vi "Host - Get Remote IO Module Data.vi"(8 "error in (no error)":errorcluster, 11 "Remote IO Mod IOVs":refnum<k21>[](array[refnum])) -> (0 "error out":errorcluster, 3 "Modules":T1[](array[typedef]))   [LabVIEW 2015, in "Scan Engine Custom Device.lvlib"]
uses:
  Scan Engine Custom Device.lvlib
  Type Defs/Host - Module.ctl
  <resource>/objmgr/IndComECAT.rc
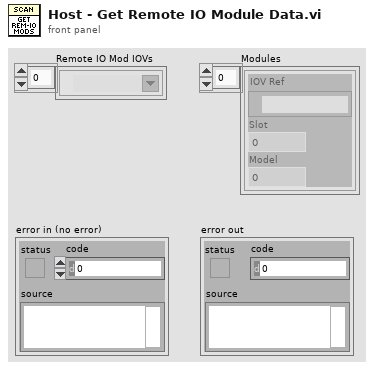
[diagram p1: front panel]
types:
  T1 = typedef "Scan Engine Custom Device.lvlib/Host - Module.ctl" = cluster{"IOV Ref":refnum<k21>, "Slot":u32, "Model":u32}
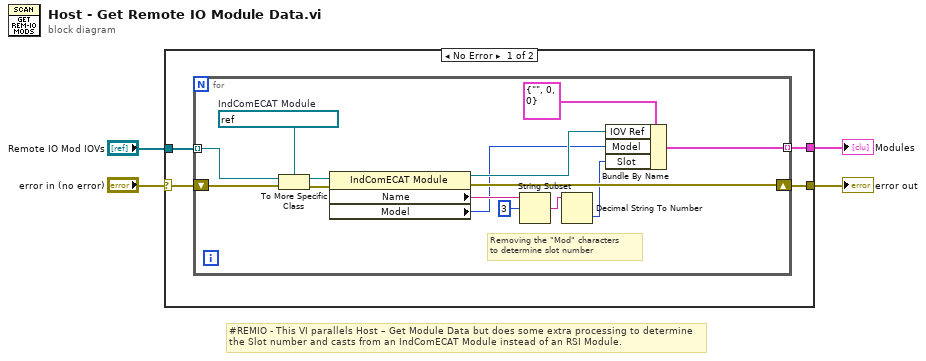
[diagram p0: block diagram]
diagram:
  # "#REMIO - This VI parallels Host – Get Module Data but does some extra processing to determine the Slot number and casts from an IndComECAT Module instead of an RSI Module."
  n1 = case shown="No Error" "error in (no error)" {
    selector: "error in (no error)" -> [w6 w23]
    tunnel: [w8 _] -> w4
    tunnel: [w7 w23] -> w3
    tunnel: "Remote IO Mod IOVs" -> [w5 _]
    frame No Error {
      n2 = for {
        shift-right: [w14] -> w7
        shift-left: w6 -> [w13]
        tunnel: [w22] -> w8 mode=indexing
        tunnel: w5 -> [w16] mode=indexing
        w15 = refnum<k21> refnum  # IndComECAT Module
        # "Removing the \"Mod\" characters\nto determine slot number"
        n3 = To More Specific Class(target class=w15, reference=w16, error in=w13) -> (specific class reference=w11:refnum<k21>, error out=w12:errorcluster)
        n4 = property class="IndComECAT Module"(reference=w11, error in=w12) -> (reference out=w17:refnum<k21>, error out=w14:errorcluster, "Name"=w20:string, "Model"=w9:u32)
        n5 = String Subset(string=w20, offset (0)=3) -> (substring=w18:string)  [unwired: 1 in]
        n6 = Decimal String To Number(string=w18) -> (number=w10:i32)  [unwired: 2 in, 1 out]
        n7 = Bundle By Name(cluster=T1 {"IOV Ref"="", "Slot"=0, "Model"=0} ("Module"), "IOV Ref"=w17, "Model"=w9, "Slot"=w10) -> (w22:T1)
      }
    }
    frame Error {
    }
  }
  "Modules" <- w4
  "error out" <- w3
